vi "SNAP_PHOTO.vi"(10 "Session Out":T1, 11 "Boolean":bool) -> (3 "Numeric 2":i32)   [LabVIEW 2015]
uses:
  <vilib>/userdefined/High Color/IMAQdx.ctl
  <vilib>/vision/driver/NI_Vision_Acquisition_Software.lvlib
panel:
  in  "Boolean 3":bool
  in  "Numeric":i32
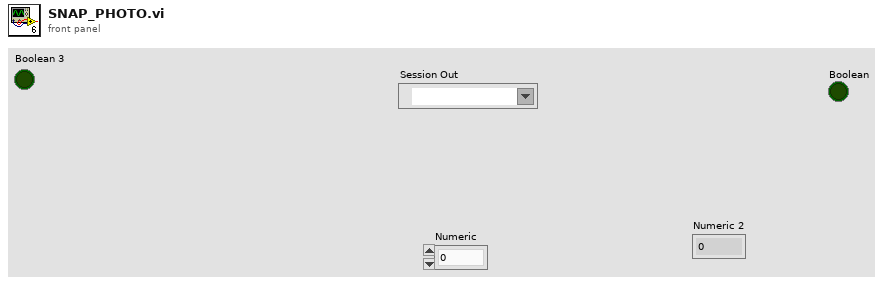
[diagram p1: front panel]
types:
  T1 = typedef "IMAQdx.ctl" = refnum<k21>
  T2 = typedef "IMAQ Image.ctl" = refnum<image>
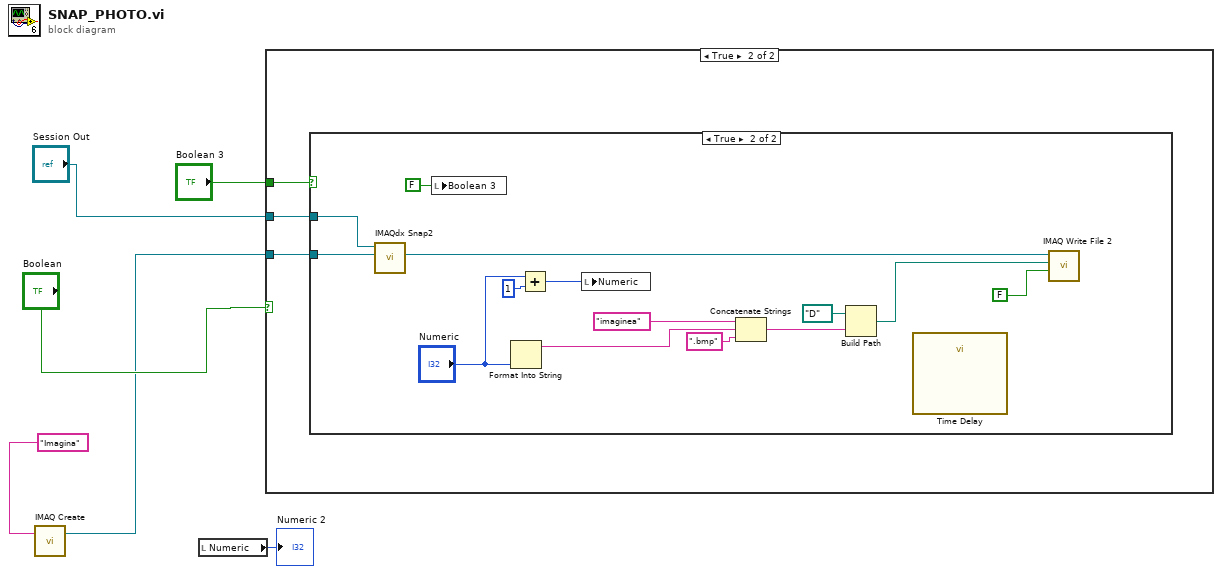
[diagram p0: block diagram]
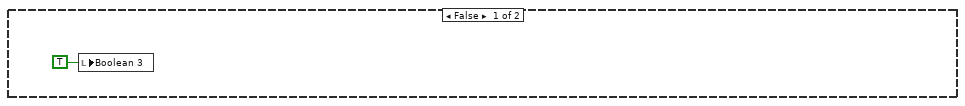
[diagram p2: hidden frame]
diagram:
  n1 = call "IMAQ Create"("Image Name"="Imagina") -> ("New Image"=w3:T2)  [unwired: 4 in, 1 out]
  n2 = local read "Numeric"() -> (→"Numeric 2":i32)
  n3 = case shown="True" "Boolean" {
    tunnel: "Boolean 3" -> [_ w10]
    tunnel: "Session Out" -> [_ w9]
    tunnel: w3 -> [_ w8]
    frame False {
      n4 = local write "Boolean 3"(TRUE) -> ()
    }
    frame True {
      n5 = case shown="True" w10 {
        tunnel: w9 -> [_ w23]
        tunnel: w8 -> [_ w22]
        frame False {
        }
        frame True {
          n6 = call <vilib>:"IMAQdx Snap2.vi"("Image In"=w22, "Session In"=w23) -> ("Image Out"=w17:T2)  [unwired: 7 in, 2 out]
          n7 = local write "Boolean 3"(FALSE) -> ()
          n8 = Format Into String("Numeric") -> (resulting string=w20:string)  [unwired: 3 in, 1 out]
          n9 = Add(x="Numeric", y=1) -> (x+y=w13:i32)
          n10 = local write "Numeric"(w13) -> ()
          n11 = Concatenate Strings("imaginea" ("string"), w20, ".bmp" ("string")) -> (w18:string)
          n12 = Build Path(base path=path "D:/", name or relative path=w18) -> (appended path=w16:path)
          n13 = call "Time Delay"() -> ()  [unwired: 11 in, 1 out]
          n14 = call-poly "IMAQ Write File 2"("Compress? (N)"=FALSE, "File Path"=w16, "Image"=w17) -> ()  [unwired: 7 in, 2 out]
        }
      }
    }
  }
